vi "Build Path.vi"(1 "To Location":cdb, 2 "Move":T1) -> (0 "Path":T2)   [LabVIEW 2020, in "AoC 2022.lvlib"]
uses:
  AoC 2022.lvlib
  Direction.ctl
  Path.ctl
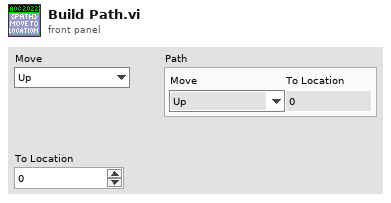
[diagram p1: front panel]
types:
  T1 = typedef "AoC 2022.lvlib/Direction.ctl" = enum16{"Up", "UpRight", "Right", "DownRight", "Down", "DownLeft", "Left", "UpLeft", "Stay"}
  T2 = typedef "AoC 2022.lvlib/Path.ctl" = cluster{"Move":T1, "To Location":cdb}
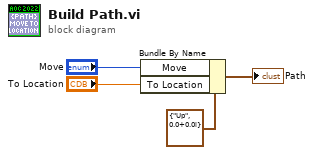
[diagram p0: block diagram]
diagram:
  n1 = Bundle By Name(cluster=T2 {"Move"=enum."Up", "To Location"=0.0+0.0i} ("Path"), "Move"="Move", "To Location"="To Location") -> (→"Path":T2)
